vi "Ctor.vi"(8 "error in (no error)":errorcluster, 11 "Terminal in":refnum<class "Terminal.lvclass">) -> (0 "error out":errorcluster, 3 "Terminal out":refnum<class "Terminal.lvclass">)   [LabVIEW 2020, in "Terminal.lvlib" / "Terminal.lvclass"]
uses:
  Terminal.lvclass
  Ref Data.ctl
  <vilib>/IlluminatedG/lv-stream/Connection/Connection.lvclass
  Parse State.ctl
  Buffer State.ctl
  Cursor.ctl
  Position.ctl
  Text Attributes.ctl
  Terminal Options.ctl
  Color Scheme.ctl
  Color.ctl
  Font Metrics.ctl
  Terminal.lvclass/Terminal.ctl
  <vilib>/IlluminatedG/IG OOPanel/OOPanel/Panel/Panel.lvclass
  Terminal.lvlib
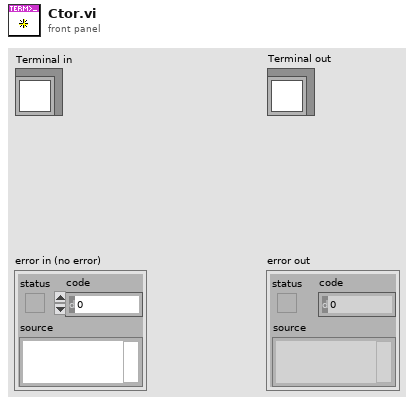
[diagram p1: front panel]
types:
  T1 = typedef "Terminal.lvlib/Terminal.lvclass/Ref Data.ctl" = cluster{"Connection":refnum<class "Connection.lvclass">, "Read Loop Running":bool, "Parse State":T2, "Terminal Options":T7, "Font Metrics":T10}
  T2 = typedef "Terminal.lvlib/Terminal.lvclass/Parse State.ctl" = cluster{"Buffer State":T3, "Cursor":T4, "Attributes":T6}
  T3 = typedef "Terminal.lvlib/Terminal.lvclass/Buffer State.ctl" = cluster{"Sequence":string, "ESC":bool, "Alt Buf":bool}
  T4 = typedef "Terminal.lvlib/Terminal.lvclass/Cursor.ctl" = cluster{"Cur":T5, "Saved":T5}
  T5 = typedef "Terminal.lvlib/Terminal.lvclass/Position.ctl" = cluster{"Row":i32, "Col":i32}
  T6 = typedef "Terminal.lvlib/Text Attributes.ctl" = cluster{"FG":u32, "BG":u32, "Bold":bool, "Italic":bool, "Underline":bool, "Strike":bool, "Inverse":bool}
  T7 = typedef "Terminal.lvlib/Terminal Options.ctl" = cluster{"Implied CR with LF":bool, "Local Echo":bool, "Tab Width":i32, "Color Scheme":T8, "Default FG":T9, "Default BG":T9, "History Length":i32, "Font Face":string, "Font Size":i16, "Rows":i32, "Cols":i32}
  T8 = typedef "Terminal.lvlib/Color Scheme.ctl" = cluster{"Black":u32, "Red":u32, "Green":u32, "Yellow":u32, "Blue":u32, "Magenta":u32, "Cyan":u32, "White":u32, "Bright Black":u32, "Bright Red":u32, "Bright Green":u32, "Bright Yellow":u32, "Bright Blue":u32, "Bright Magenta":u32, "Bright Cyan":u32, "Bright White":u32}
  T9 = typedef "Terminal.lvlib/Color.ctl" = i8
  T10 = typedef "Terminal.lvlib/Terminal.lvclass/Font Metrics.ctl" = cluster{"Width":i16, "Height":i16}
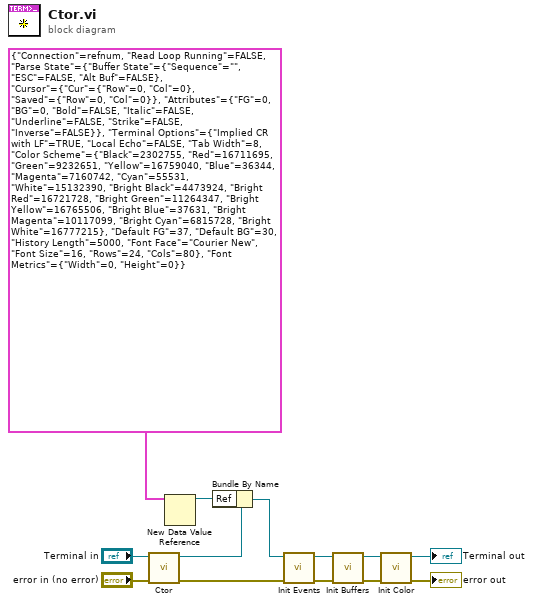
[diagram p0: block diagram]
diagram:
  n1 = call-parent "Ctor.vi"("error in (no error)"="error in (no error)", "Panel in"="Terminal in") -> ("error out"=w8:errorcluster, "Panel out"=w9:refnum<class "Terminal.lvclass">)  [unwired: 8 in]
  n2 = New Data Value Reference(data value=T1 {"Connection"=refnum, "Read Loop Running"=FALSE, "Parse State"={"Buffer State"={"Sequence"="", "ESC"=FALSE, "Alt Buf"=FALSE}, "Cursor"={"Cur"={"Row"=0, "Col"=0}, "Saved"={"Row"=0, "Col"=0}}, "Attributes"={"FG"=0, "BG"=0, "Bold"=FALSE, "Italic"=FALSE, "Underline"=FALSE, "Strike"=FALSE, "Inverse"=FALSE}}, "Terminal Options"={"Implied CR with LF"=TRUE, "Local Echo"=FALSE, "Tab Width"=8, "Color Scheme"={"Black"=2302755, "Red"=16711695, "Green"=9232651, "Yellow"=16759040, "Blue"=36344, "Magenta"=7160742, "Cyan"=55531, "White"=15132390, "Bright Black"=4473924, "Bright Red"=16721728, "Bright Green"=11264347, "Bright Yellow"=16765506, "Bright Blue"=37631, "Bright Magenta"=10117099, "Bright Cyan"=6815728, "Bright White"=16777215}, "Default FG"=37, "Default BG"=30, "History Length"=5000, "Font Face"="Courier New", "Font Size"=16, "Rows"=24, "Cols"=80}, "Font Metrics"={"Width"=0, "Height"=0}} ("Ref Data")) -> (data value reference=w12:refnum<data-value>)  [unwired: 1 in, 1 out]
  n3 = Bundle By Name(cluster=w9, "Ref"=w12) -> (w7:refnum<class "Terminal.lvclass">)
  n4 = call "Init Events.vi"("error in (no error)"=w8, "Terminal in"=w7) -> ("error out"=w6:errorcluster, "Terminal out"=w5:refnum<class "Terminal.lvclass">)  [unwired: 8 in]
  n5 = call "Init Buffers.vi"("error in (no error)"=w6, "Terminal in"=w5) -> ("error out"=w3:errorcluster, "Terminal out"=w4:refnum<class "Terminal.lvclass">)  [unwired: 8 in]
  n6 = call "Init Color.vi"("error in (no error)"=w3, "Terminal in"=w4) -> ("error out"=→"error out":errorcluster, "Terminal out"=→"Terminal out":refnum<class "Terminal.lvclass">)  [unwired: 8 in]
